vi "Emballage_BDD_lecture_Table_Correspondance.vi"(8 "entrée d'erreur (pas d'erreur)":errorcluster, 11 "Famille":string) -> (0 "error out":errorcluster, 2 "Result Set":string[][](table) caption="Result Set (from first statement with results)", 3 "Column Names":string[](array[string]))   [LabVIEW 2020]
uses:
  Modules/FS/60_FS_Controles/60_FS_SetGet.ctl
  <vilib>/addons/database/Connection.llb/DB Tools Open Connec (Path).vi
  <vilib>/addons/database/Connection.llb/Conn Execute.vi
  <vilib>/addons/database/Recordset.llb/Rec Fetch Recordset Data (R).vi
  <vilib>/addons/database/Recordset.llb/Rec Destroy - Connection.vi
  <vilib>/addons/database/NI_Database_API.lvlib
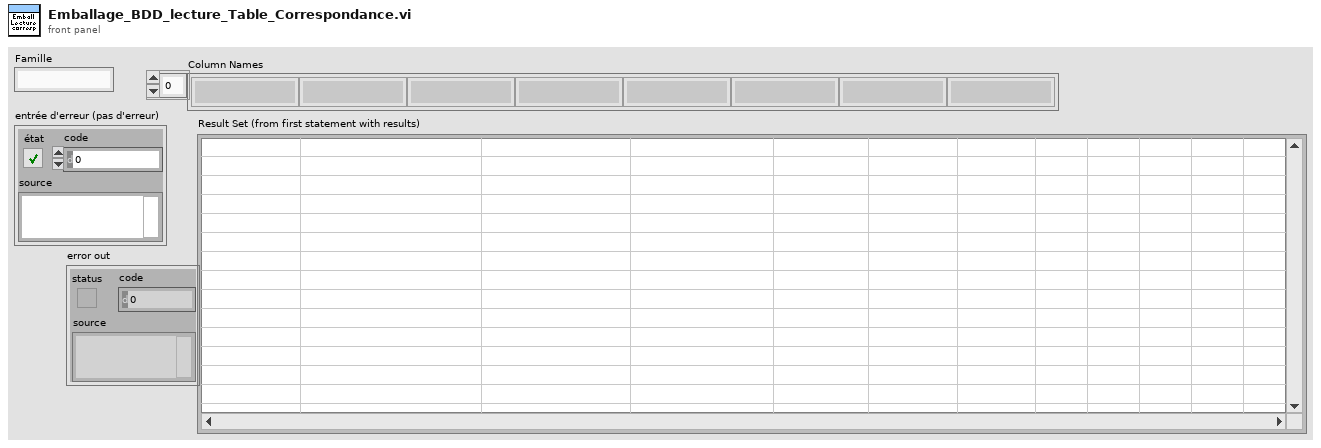
[diagram p1: front panel]
types:
  T1 = typedef "60_FS_SetGet.ctl" = enum16{"set", "get"}
  T2 = typedef "60_FS_CLT_Chemins.ctl" = cluster{"Racine_local":path, "Racine_reseau":path, "Racine_Support_Application":path, "Fichier_Journalisation":path, "Connexion_BDD_VSX":path, "Connexion_BDD_PLZ":path}
  T3 = typedef "NI_Database_API.lvlib/Conn ObjectReference.ctl" = refnum<k1>
  T4 = typedef "NI_Database_API.lvlib/Rec ObjectReference.ctl" = refnum<k1>
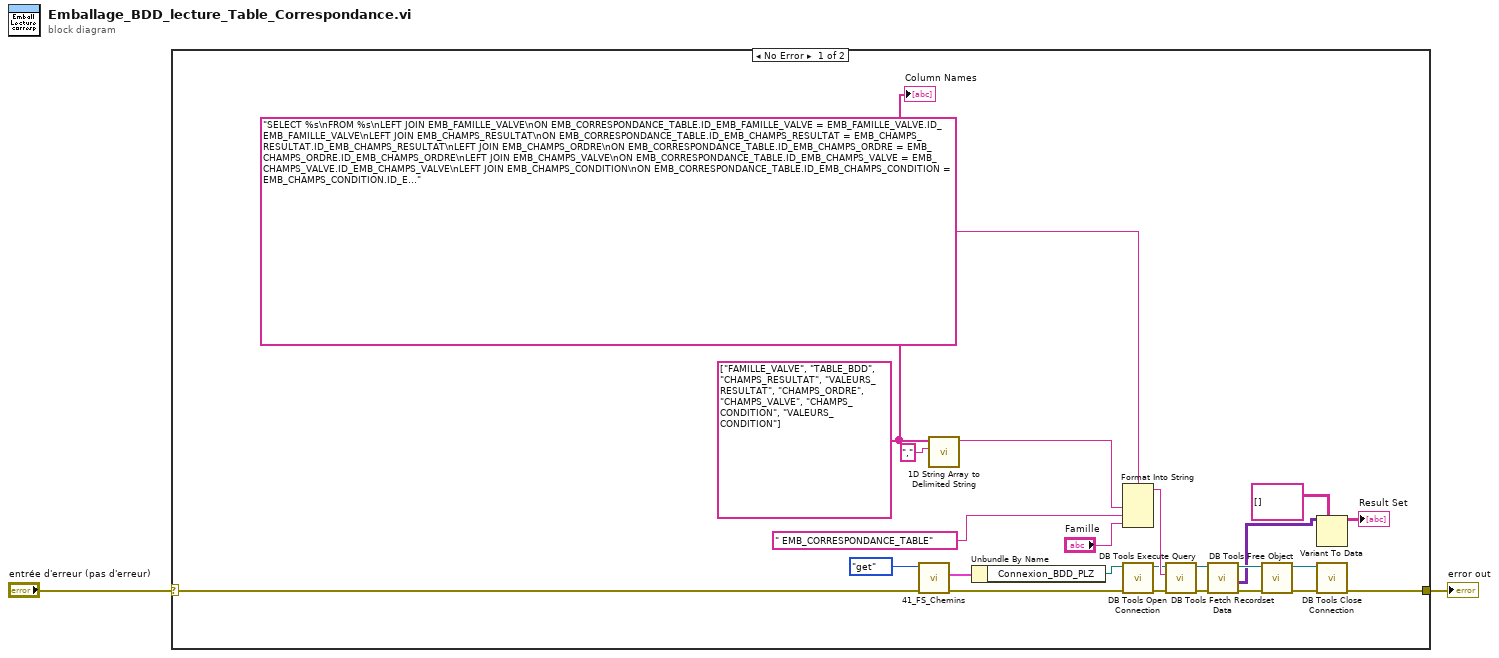
[diagram p0: block diagram]
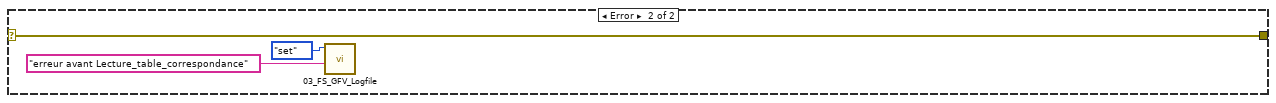
[diagram p2: hidden frame]
diagram:
  n1 = case shown="No Error" "entrée d'erreur (pas d'erreur)" {
    selector: "entrée d'erreur (pas d'erreur)" -> [w7 w29]
    tunnel: [w6 w29] -> w1
    frame No Error {
      w3 = string[] ["FAMILLE_VALVE", "TABLE_BDD", "CHAMPS_RESULTAT", "VALEURS_RESULTAT", "CHAMPS_ORDRE", "CHAMPS_VALVE", "CHAMPS_CONDITION", "VALEURS_CONDITION"]
      n2 = call "41_FS_Chemins.vi"("error in (no error)"=w7, "SetGet"=60_FS_SetGet."get") -> ("error out"=w16:errorcluster, "CLT_Chemins_out"=w24:T2)  [unwired: 8 in]
      n3 = call <vilib>:"1D String Array to Delimited String.vi"("delimiter"=",", "string array"=w3) -> ("delimited string"=w5:string)  [unwired: 9 in]
      n4 = Unbundle By Name(w24) -> ("Connexion_BDD_PLZ"=w17:path)
      n5 = Format Into String(format string="SELECT %s\nFROM %s\nLEFT JOIN EMB_FAMILLE_VALVE\nON EMB_CORRESPONDANCE_TABLE.ID_EMB_FAMILLE_VALVE = EMB_FAMILLE_VALVE.ID_EMB_FAMILLE_VALVE\nLEFT JOIN EMB_CHAMPS_RESULTAT\nON EMB_CORRESPONDANCE_TABLE.ID_EMB_CHAMPS_RESULTAT = EMB_CHAMPS_RESULTAT.ID_EMB_CHAMPS_RESULTAT\nLEFT JOIN EMB_CHAMPS_ORDRE\nON EMB_CORRESPONDANCE_TABLE.ID_EMB_CHAMPS_ORDRE = EMB_CHAMPS_ORDRE.ID_EMB_CHAMPS_ORDRE\nLEFT JOIN EMB_CHAMPS_VALVE\nON EMB_CORRESPONDANCE_TABLE.ID_EMB_CHAMPS_VALVE = EMB_CHAMPS_VALVE.ID_EMB_CHAMPS_VALVE\nLEFT JOIN EMB_CHAMPS_CONDITION\nON EMB_CORRESPONDANCE_TABLE.ID_EMB_CHAMPS_CONDITION = EMB_CHAMPS_CONDITION.ID_EMB_CHAMPS_CONDITION\nLEFT JOIN EMB_VALEURS_CONDITION\nON EMB_CORRESPONDANCE_TABLE.ID_EMB_VALEURS_CONDITION = EMB_VALEURS_CONDITION.ID_EMB_VALEURS_CONDITION\nWHERE EMB_FAMILLE_VALVE.FAMILLE_VALVE = '%s'" ("SQL"), w5, " EMB_CORRESPONDANCE_TABLE" ("table"), "Famille") -> (resulting string=w15:string)  [unwired: 2 in, 1 out]
      n6 = call-poly <vilib>:"DB Tools Open Connection.vi"("error in (no error)"=w16, "connection information"=w17) -> ("error out"=w12:errorcluster, "connection reference"=w9:T3)  [unwired: 6 in]
      n7 = call-poly <vilib>:"DB Tools Execute Query.vi"("error in (no error)"=w12, "SQL query"=w15, "connection reference"=w9) -> ("error out"=w21:errorcluster, "recordset reference"=w19:T4)  [unwired: 5 in]
      n8 = call-poly <vilib>:"DB Tools Fetch Recordset Data.vi"("error in (no error)"=w21, "recordset reference"=w19) -> ("error out"=w20:errorcluster, "recordset data"=w13:variant[][], "recordset reference out"=w18:T4)  [unwired: 3 in]
      n9 = call-poly <vilib>:"DB Tools Free Object.vi"("error in (no error)"=w20, "recordset reference"=w18) -> ("error out"=w23:errorcluster, "connection reference"=w22:T3)  [unwired: 8 in]
      n10 = Variant To Data(type=string[][] [] ("Liste des champs à lire 2"), Variant=w13) -> (data=→"Result Set":string[][])  [unwired: 1 in, 1 out]
      n11 = call <vilib>:"DB Tools Close Connection.vi"("error in (no error)"=w23, "connection reference"=w22) -> ("error out"=w6:errorcluster)  [unwired: 5 in]
      "Column Names" <- w3
    }
    frame Error {
      n12 = call "03_FS_GFV_Logfile.vi"("Chaîne"="erreur avant Lecture_table_correspondance", "States"=60_FS_SetGet."set") -> ()  [unwired: 8 in, 2 out]
    }
  }
  "error out" <- w1
